vi "Culab Not Complex Process.vi"(11 "X size":i32=16384) -> (3 "Culab Time":dbl=1.016902899999991)   [LabVIEW 2020]
uses:
  <vilib>/Ngene/CuLab - GPU Accelerated Toolkit/Toolkit/Low_Level/Tensor_Classes/T_Children/T1D/T1D_Children/T1D_SGL/Create_Push.vi
  <vilib>/Ngene/CuLab - GPU Accelerated Toolkit/Toolkit/Low_Level/Tensor_Classes/T_Children/T0D/T0D_Children/T0D_SGL/Create.vi
  <vilib>/Ngene/CuLab - GPU Accelerated Toolkit/Toolkit/Low_Level/Tensor_Classes/T_Children/T0D/T0D_Children/T0D_SGL/Pull.vi
  <vilib>/Ngene/CuLab - GPU Accelerated Toolkit/Toolkit/CuLab.lvlib
  <vilib>/Ngene/CuLab - GPU Accelerated Toolkit/Toolkit/Low_Level/Tensor_Classes/T_Children/T0D/T0D_Children/T0D_SGL/T0D_SGL.lvclass
  <vilib>/Ngene/CuLab - GPU Accelerated Toolkit/Toolkit/Low_Level/Tensor_Classes/T_Children/T1D/T1D_Children/T1D_SGL/T1D_SGL.lvclass
  <vilib>/Analysis/NI_AALBase.lvlib
panel:
  out "Dest out":sgl=7.867303e+19
  in  "nb_loop":i32=6
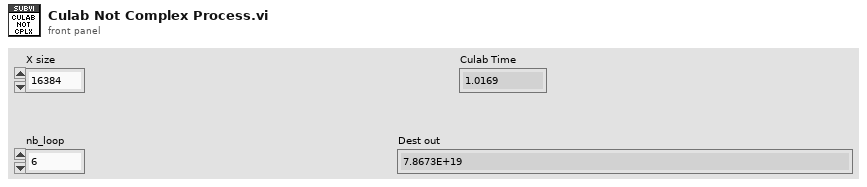
[diagram p1: front panel]
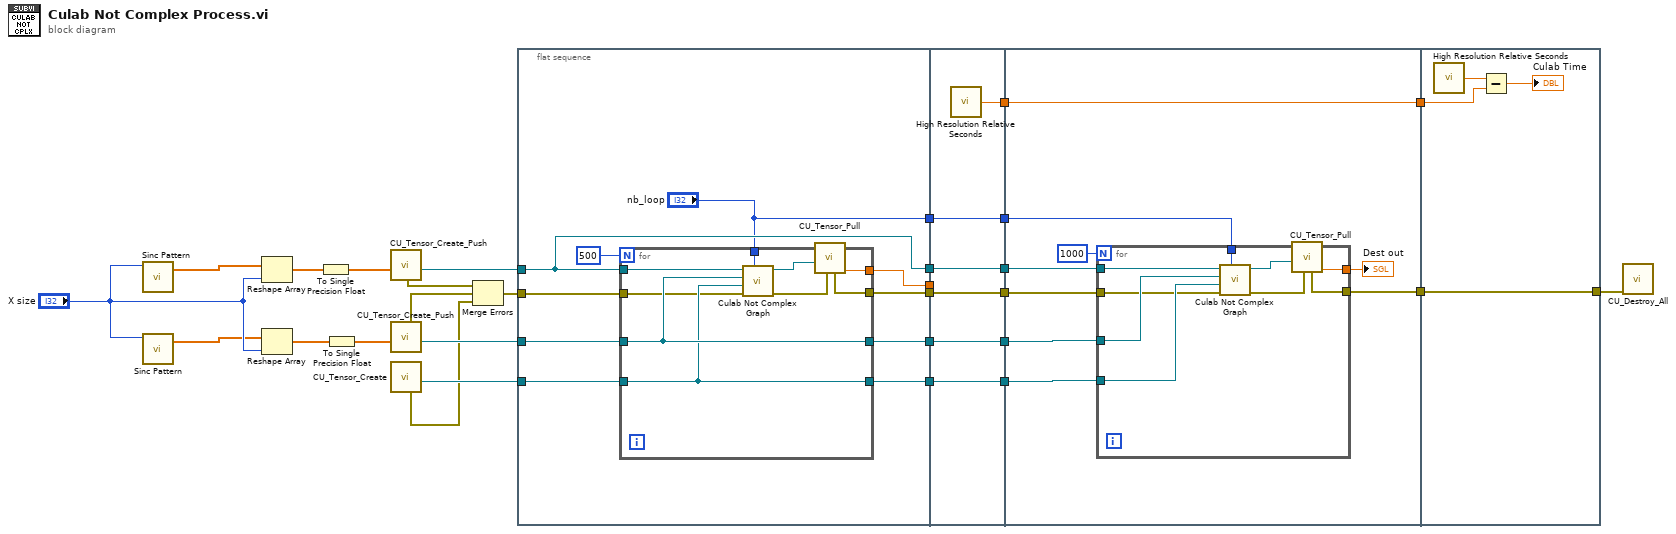
[diagram p0: block diagram]
diagram:
  n1 = call <vilib>:"Sinc Pattern.vi"("samples"="X size") -> ("Sinc Pattern"=w2:dbl[])  [unwired: 3 in, 1 out]
  n2 = call <vilib>:"Sinc Pattern.vi"("samples"="X size") -> ("Sinc Pattern"=w1:dbl[])  [unwired: 3 in, 1 out]
  n3 = Reshape Array(w2, "X size") -> (w10:dbl[])
  n4 = Reshape Array(w1, "X size") -> (w9:dbl[])
  n5 = To Single Precision Float(number=w10) -> (single precision float=w8:sgl[])
  n6 = To Single Precision Float(number=w9) -> (single precision float=w7:sgl[])
  n7 = call-poly <vilib>:"CU_Tensor_Create_Push.vi"("CPU_Data_1D_SGL"=w8) -> ("T1D_SGL out"=w26:refnum<class "T1D_SGL.lvclass">, "error out"=w4:errorcluster)  [unwired: 9 in]
  n8 = call-poly <vilib>:"CU_Tensor_Create_Push.vi"("CPU_Data_1D_SGL"=w7) -> ("T1D_SGL out"=w25:refnum<class "T1D_SGL.lvclass">, "error out"=w5:errorcluster)  [unwired: 9 in]
  n9 = call-poly <vilib>:"CU_Tensor_Create.vi"() -> ("T0D_SGL out"=w24:refnum<class "T0D_SGL.lvclass">, "error out"=w6:errorcluster)  [unwired: 10 in]
  n10 = Merge Errors(w4, w5, w6) -> (w3:errorcluster)
  n11 = flat-sequence {
    tunnel: w24 -> [w34]
    tunnel: w25 -> [w39]
    tunnel: w26 -> [w37]
    tunnel: [w38] -> w23
    tunnel: [w37] -> w22
    tunnel: [w35] -> w20
    tunnel: [w33] -> w18
    tunnel: [w32] -> w16
    tunnel: ["nb_loop"] -> w12
    tunnel: w3 -> [w30]
    tunnel: [w54] -> w29
    tunnel: [w53] -> w28
    tunnel: w23 -> [_]
    tunnel: w22 -> [w53]
    tunnel: [w52] -> w21
    tunnel: w20 -> [w52]
    tunnel: [w51] -> w19
    tunnel: w18 -> [w51]
    tunnel: [w50] -> w17
    tunnel: w16 -> [w50]
    tunnel: [w49] -> w13
    tunnel: w12 -> [w49]
    tunnel: w29 -> [w63]
    tunnel: [w63] -> w27
    tunnel: w28 -> [w60]
    tunnel: w21 -> [w56]
    tunnel: w19 -> [w62]
    tunnel: w17 -> [w61]
    tunnel: [w58] -> w14
    tunnel: w13 -> [w57]
    tunnel: w27 -> [w75]
    tunnel: [w73] -> w15
    tunnel: w14 -> [w73]
    frame #0 {
      n12 = for {
        N: 500 -> [_]
        tunnel: w39 -> [w44]
        tunnel: [w48] -> w38
        tunnel: w37 -> [w46]
        tunnel: [w47] -> w35
        tunnel: w34 -> [w43]
        tunnel: [w44] -> w33
        tunnel: [w43] -> w32
        tunnel: "nb_loop" -> [w42]
        tunnel: w30 -> [w40]
        n13 = call "Culab Not Complex Graph.vi"("nb_loop"=w42, "error in (no error)"=w40, "C"=w43, "B"=w44, "A"=w46) -> ("error out"=w41:errorcluster, "Dest out"=w45:refnum<class "T0D_SGL.lvclass">)  [unwired: 5 in]
        n14 = call-poly <vilib>:"CU_Tensor_Pull.vi"("error in (no error)"=w41, "T0D_SGL in"=w45) -> ("Dest out"=w48:sgl, "error out"=w47:errorcluster)  [unwired: 7 in, 1 out]
      }
    }
    frame #1 {
      n15 = call <vilib>:"High Resolution Relative Seconds.vi"() -> ("relative seconds"=w54:dbl)
    }
    frame #2 {
      n16 = for {
        N: 1000 -> [_]
        tunnel: w62 -> [w69]
        tunnel: [w72] -> w55
        tunnel: w60 -> [w70]
        tunnel: [w71] -> w58
        tunnel: w61 -> [w67]
        tunnel: w57 -> [w66]
        tunnel: w56 -> [w65]
        n17 = call "Culab Not Complex Graph.vi"("nb_loop"=w66, "error in (no error)"=w65, "C"=w67, "B"=w69, "A"=w70) -> ("error out"=w64:errorcluster, "Dest out"=w68:refnum<class "T0D_SGL.lvclass">)  [unwired: 5 in]
        n18 = call-poly <vilib>:"CU_Tensor_Pull.vi"("error in (no error)"=w64, "T0D_SGL in"=w68) -> ("Dest out"=w72:sgl, "error out"=w71:errorcluster)  [unwired: 7 in, 1 out]
      }
      "Dest out" <- w55
    }
    frame #3 {
      n19 = call <vilib>:"High Resolution Relative Seconds.vi"() -> ("relative seconds"=w76:dbl)
      n20 = Subtract(x=w76, y=w75) -> (x-y=→"Culab Time":dbl)
    }
  }
  n21 = call <vilib>:"CU_Destroy_All.vi"("error in"=w15) -> ()  [unwired: 10 in, 1 out]
